vi "send error.vi"(8 "error in (no error)":errorcluster, 9 "Queues":refnum<queue>[](array[refnum]), 10 "System Data":T1, 11 "Last State":string) -> ()   [LabVIEW 2017]
uses:
  Queue Element.ctl
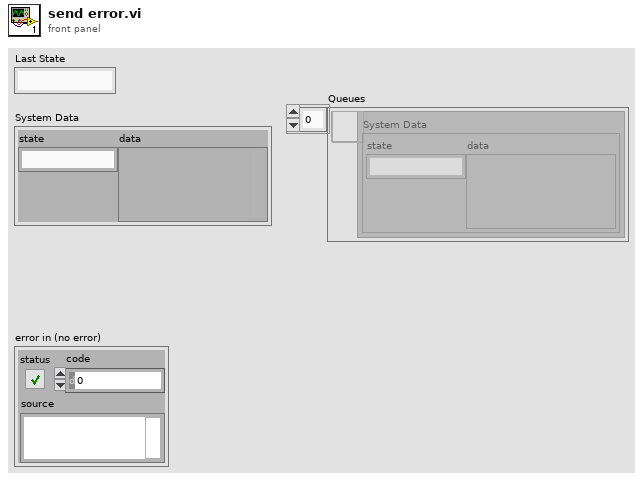
[diagram p1: front panel]
types:
  T1 = typedef "Queue Element.ctl" = cluster{"state":string, "data":variant}
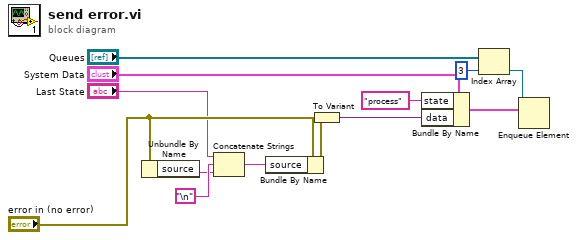
[diagram p0: block diagram]
diagram:
  n1 = Unbundle By Name("error in (no error)") -> ("source"=w8:string)
  n2 = Concatenate Strings("Last State", "\n", w8) -> (w11:string)
  n3 = Bundle By Name(cluster="error in (no error)", "source"=w11) -> (w13:errorcluster)
  n4 = To Variant(anything=w13) -> (Variant=w7:variant)
  n5 = Bundle By Name(cluster="System Data", "state"="process", "data"=w7) -> (w4:T1)
  n6 = Index Array(array="Queues", index=3) -> (element=w3:refnum<queue>)
  n7 = Enqueue Element(queue=w3, element=w4) -> ()  [unwired: 2 in, 3 out]
